vi "Set General Queue Array Element.vi"(8 "error in (no error)":errorcluster, 10 "array in":T1[](array[typedef])=[enum."initialise ueye camera", enum."initialise standa motor", enum."initialise position motor"], 11 "queue in":refnum<queue>) -> (0 "error out":errorcluster, 3 "queue out":refnum<queue>)   [LabVIEW 2010, in "SignalWriterMH110203USBStepperMotor.lvclass"]
uses:
  SignalWriterMH110203USBStepperMotor.lvclass
  event_controller.ctl
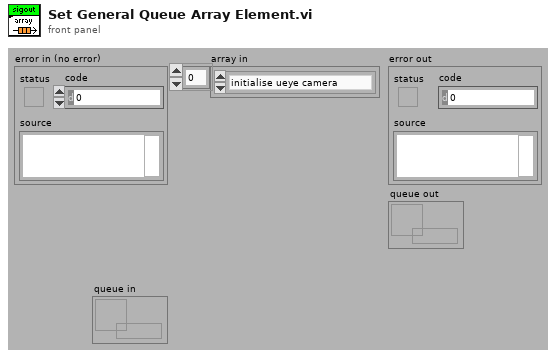
[diagram p1: front panel]
types:
  T1 = typedef "SignalWriterMH110203USBStepperMotor.lvclass/event_controller.ctl" = enum16{"initialise ueye camera", "get new position to go", "convert ROIs", "load profile", "initialise standa motor", "change ROI", "grab frame", "set binning", "invert image", "get position standa motor", "initialise position motor", "go to position", "update motor speed step", "exit ueye camera", "exit standa motor"}
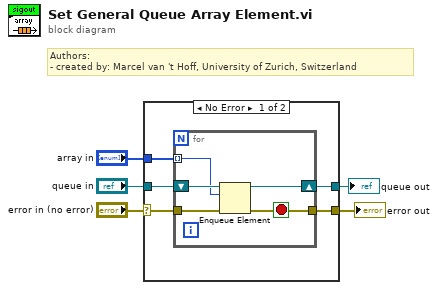
[diagram p0: block diagram]
diagram:
  # "Authors: \n- created by: Marcel van 't Hoff, University of Zurich, Switzerland"
  n1 = case shown="No Error" "error in (no error)" {
    selector: "error in (no error)" -> [w8 w17]
    tunnel: [w10 w17] -> w5
    tunnel: [w9 w16] -> w2
    tunnel: "queue in" -> [w7 w16]
    tunnel: "array in" -> [w6 _]
    frame No Error {
      n2 = for {
        tunnel: w8 -> [w12]
        tunnel: [w13] -> w10
        shift-right: [w14] -> w9
        shift-left: w7 -> [w15]
        tunnel: w6 -> [w11] mode=indexing
        stop <- w13 stop-if-true
        n3 = Enqueue Element(queue=w15, element=w11, error in (no error)=w12) -> (queue out=w14:refnum<queue>, error out=w13:errorcluster)  [unwired: 1 in, 1 out]
      }
    }
    frame Error {
    }
  }
  "error out" <- w5
  "queue out" <- w2
